vi "DINT Write.vi"(7 "stn":i32[](array[numeric]), 10 "Tag Name":string, 11 "Network Path":string) -> (2 "error out":errorcluster)   [LabVIEW 2020]
uses:
  <vilib>/ethernetip/ethernetip.llb/EthernetIP Tag Write DINT.vi
  <vilib>/ethernetip/ethernetip.lvlib
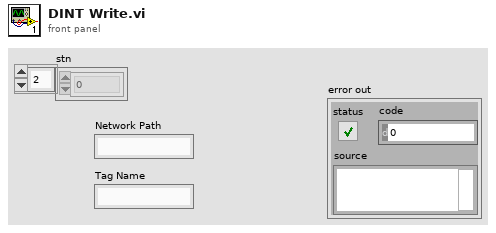
[diagram p1: front panel]
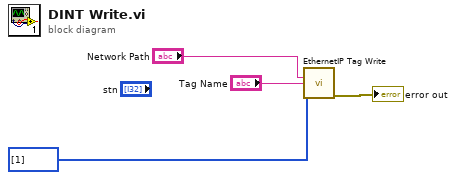
[diagram p0: block diagram]
diagram:
  n1 = call-poly <vilib>:"EthernetIP Tag Write.vi"("Network Path"="Network Path", "Tag Name"="Tag Name", "Data"=i32[] [1]) -> ("error out"=→"error out":errorcluster)  [unwired: 11 in, 1 out]
